vi "WCA_SET_PA_VG_Band10.vi"(0 "Cartridge Band":u32=10, 1 "Slave Node in":cluster{"Address":i16, "Serial Number":i8[]}={"Address"=19, "Serial Number"=[16, 71, 55, 76, 1, 8, 0, -15]} {"Serial Number" format="%.0x"; "Address" format="%.0x"}, 2 "ObjHandle in":u32, 5 "POL（P0、P1）":u32, 9 "SET_PA_VG":dbl, 11 "error in (no error)":errorcluster) -> (4 "ObjHandle out":u32=92930112, 15 "error out":errorcluster)   [LabVIEW 2017]
uses:
  WCA_Global.vi
panel:
  # "Node Address"
  # "Serial Number"
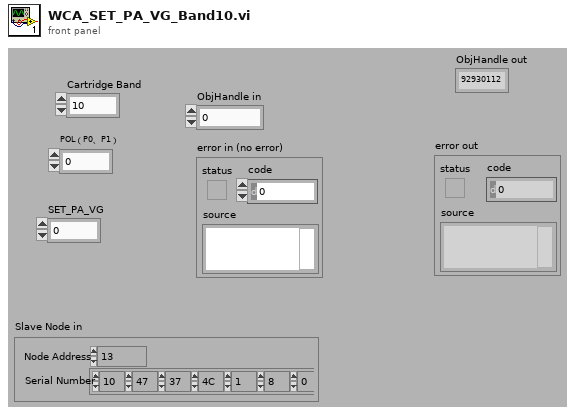
[diagram p1: front panel]
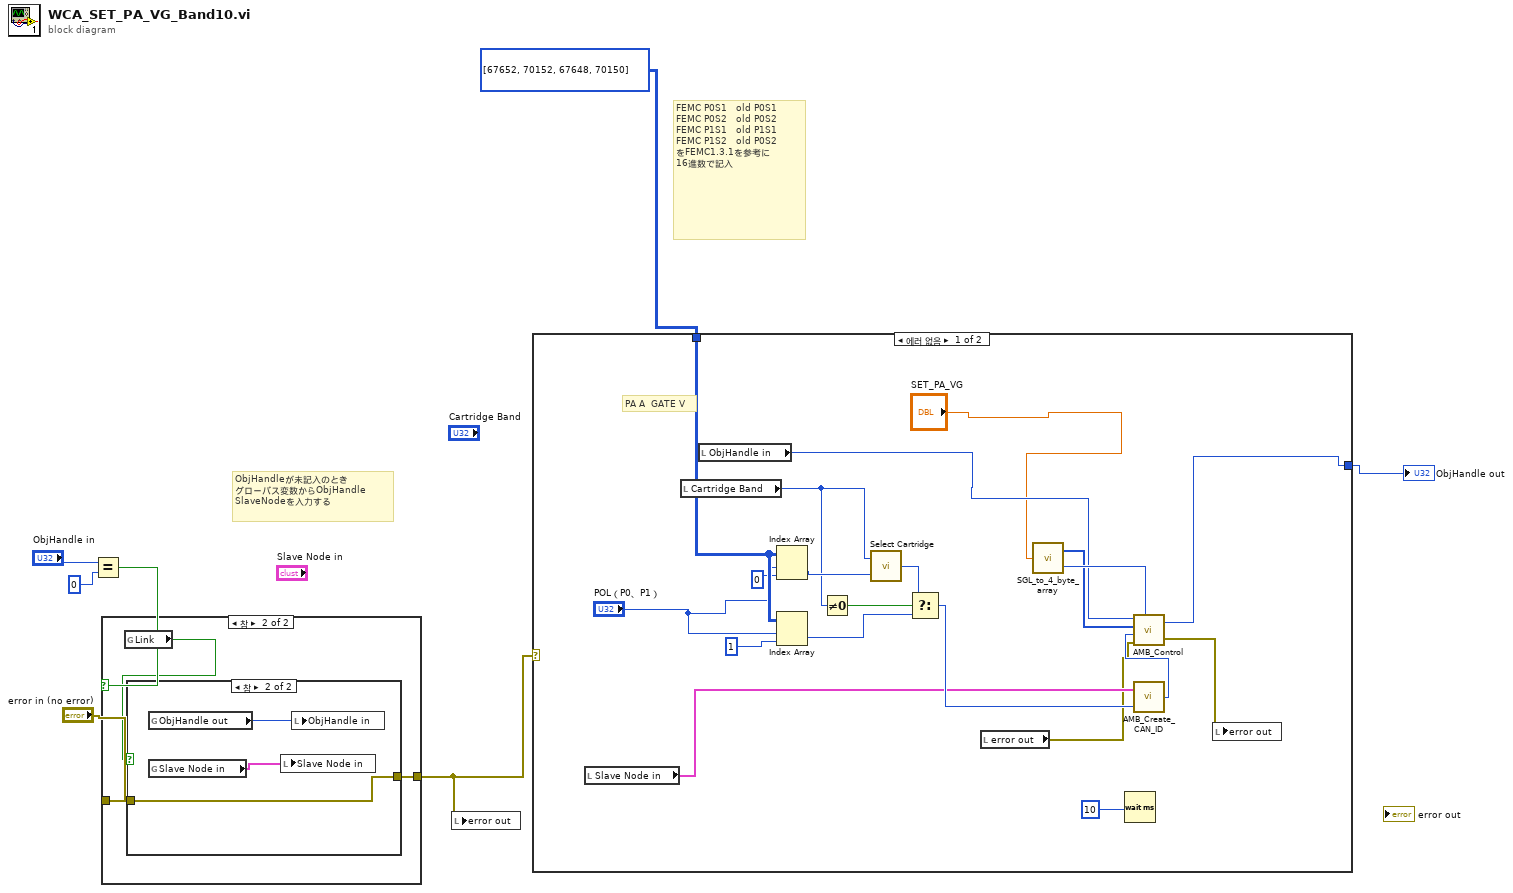
[diagram p0: block diagram]
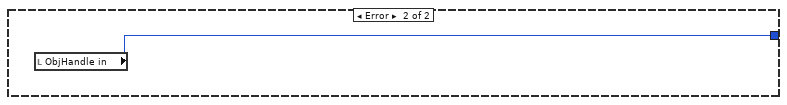
[diagram p2: hidden frame]
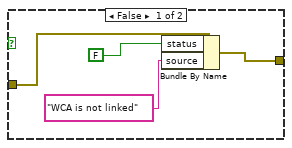
[diagram p4: hidden frame]
diagram:
  # "ObjHandleが未記入のとき\nグローバス変数からObjHandle\nSlaveNodeを入力する"
  # "FEMC P0S1   old P0S1\nFEMC P0S2   old P0S2\nFEMC P1S1   old P1S1\nFEMC P1S2   old P0S2\nをFEMC1.3.1を参考に\n16進数で記入"
  n1 = Equal?(x="ObjHandle in", y=0) -> (x = y?=w5:bool)
  n2 = case shown="참" w5 {
    tunnel: "error in (no error)" -> [w8 w11]
    tunnel: [w8 w10] -> w3
    frame False {
    }
    frame True {
      n3 = global read "WCA_Global.vi" "Link"() -> (w9:bool)
      n4 = case shown="참" w9 {
        tunnel: w11 -> [w15 w16]
        tunnel: [w12 w16] -> w10
        frame False {
          n5 = Bundle By Name(cluster=w15, "status"=FALSE, "source"="WCA is not linked") -> (w12:errorcluster)
        }
        frame True {
          n6 = global read "WCA_Global.vi" "ObjHandle out"() -> (w18:u32)
          n7 = global read "WCA_Global.vi" "Slave Node in"() -> (w17:cluster{"Address":i16, "Serial Number":i8[]})
          n8 = local write "Slave Node in"(w17) -> ()
          n9 = local write "ObjHandle in"(w18) -> ()
        }
      }
    }
  }
  n10 = local write "error out"(w3) -> ()
  n11 = case shown="에러 없음" w3 {
    tunnel: [w19 w39] -> w2
    tunnel: i32[][] [[67652, 70152], [67648, 70150]] -> [w38 _]
    frame No Error {
      # "PA A  GATE V"
      n12 = local read "Slave Node in"() -> (w25:cluster{"Address":i16, "Serial Number":i8[]})
      n13 = local read "Cartridge Band"() -> (w31:u32)
      n14 = local read "ObjHandle in"() -> (w27:u32)
      n15 = Index Array(array=w38, index (row)="POL（P0、P1）", index (col)=0) -> (element=w34:i32)
      n16 = Index Array(array=w38, index (row)="POL（P0、P1）", index (col)=1) -> (element=w35:i32)
      n17 = Not Equal To 0?(x=w31) -> (x != 0?=w36:bool)
      n18 = call "Select Cartridge.vi"("Relative Address in"=w34, "Cartridge band"=w31) -> ("Relative Address out"=w37:u32)
      n19 = Select(t=w37, s=w36, f=w35) -> (s? t:f=w26:u32)
      n20 = local read "error out"() -> (w24:errorcluster)
      n21 = call "SGL_to_4_byte_array.vi"("SGL float"="SET_PA_VG") -> ("SGL float encoded array of bytes"=w28:u8[], "bytes"=w29:u32)
      n22 = Wait (ms)(milliseconds to wait=10) -> ()  [unwired: 1 out]
      n23 = call "AMB_Create_CAN_ID.vi"("Relative Address in"=w26, "Slave Node in"=w25) -> ("CAN ID out"=w30:u32)
      n24 = call "AMB_Control.vi"("ObjHandle in"=w27, "Data in"=w28, "CAN ID in"=w30, "error in"=w24, "Data Length in"=w29) -> ("ObjHandle out"=w19:u32, "error out"=w23:errorcluster)
      n25 = local write "error out"(w23) -> ()
    }
    frame Error {
      n26 = local read "ObjHandle in"() -> (w39:u32)
    }
  }
  "ObjHandle out" <- w2
